vi "SCOPE_Measure.vi"(8 "error in (no error)":errorcluster, 9 "Data Cluster":T1 {"GUI Data Cluster"."SBR" format="%08b"}, 10 "Configuration Cluster":T3={"General"={"Config.ini"=path "", "Default Logging Path"=path ""}, "Hardware"={"Global T VAR"="", "Global B VAR"="", "VISAS"={"GEN COM"="", "SCOPE COM"="", "VNA COM"=""}, "Connected?"={"SCOPE"=FALSE, "GEN"=FALSE, "VNA"=FALSE}}, "Operation"={"Operation Mode"=enum."Idle-Off", "Status"="", "NewLog?"=FALSE, "OvenWarn"=FALSE, "Scope Settings"={"TimeBase"=0.0, "VerticalScale"=4.0, "Channel"=enum."Channel 2"}, "Gen Settings"={"Amplitude"=0.0, "Frequency"=0.0, "Offset"=0.0}}}) -> (0 "error out":errorcluster, 1 "Data Cluster out":T1 {"GUI Data Cluster"."SBR" format="%08b"}, 2 "Configuration Cluster Out":T3={"General"={"Config.ini"=path "", "Default Logging Path"=path ""}, "Hardware"={"Global T VAR"="", "Global B VAR"="", "VISAS"={"GEN COM"="", "SCOPE COM"="", "VNA COM"=""}, "Connected?"={"SCOPE"=FALSE, "GEN"=FALSE, "VNA"=FALSE}}, "Operation"={"Operation Mode"=enum."Idle-Off", "Status"="", "NewLog?"=FALSE, "OvenWarn"=FALSE, "Scope Settings"={"TimeBase"=0.0, "VerticalScale"=0.0, "Channel"=enum."Channel 2"}, "Gen Settings"={"Amplitude"=0.0, "Frequency"=0.0, "Offset"=0.0}}})   [LabVIEW 2021]
uses:
  Config_Cluster.ctl
  Mode_Enum.ctl
  Data_Cluster.ctl
  Measurement_Cluster.ctl
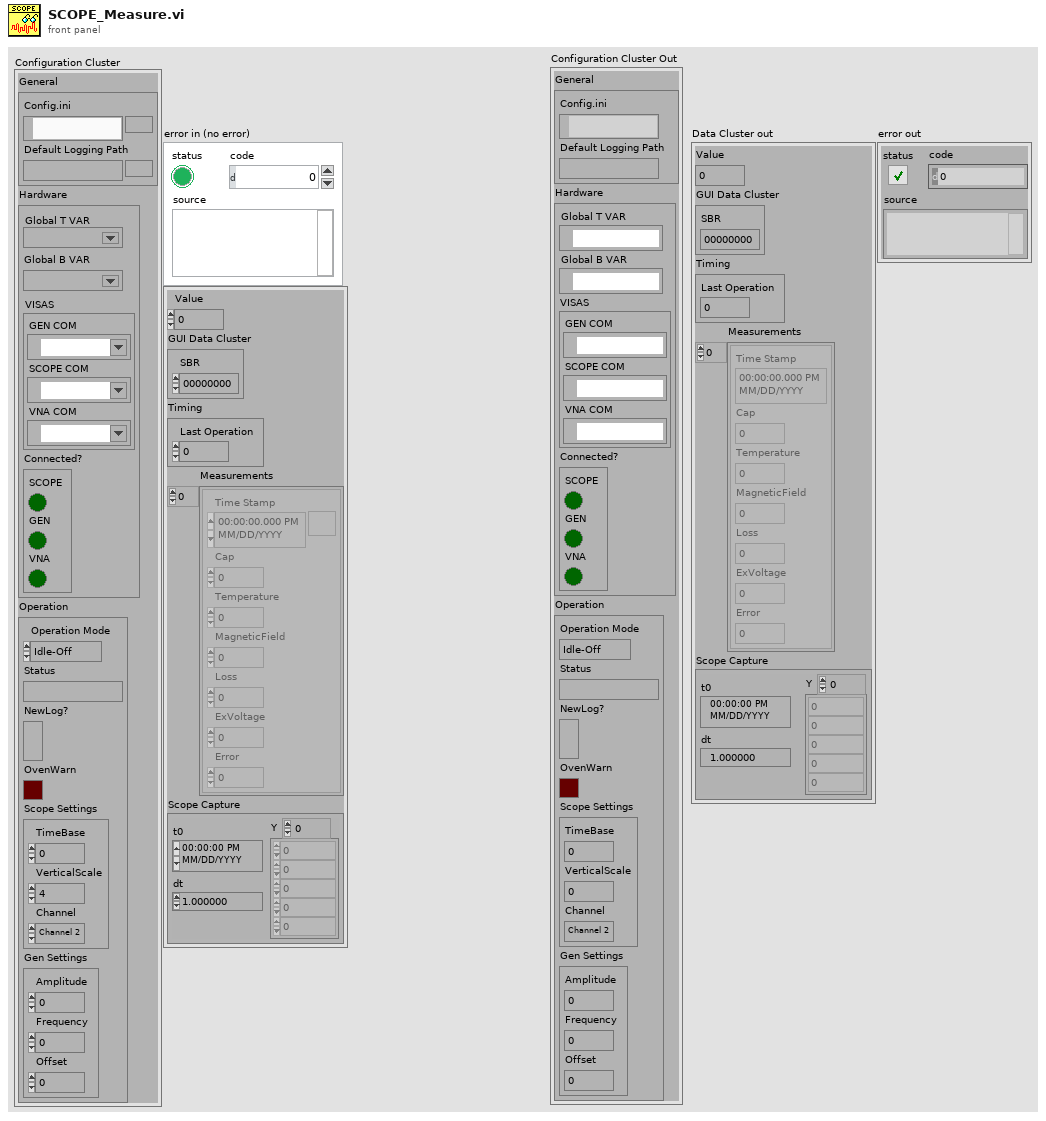
[diagram p1: front panel]
types:
  T1 = typedef "Data_Cluster.ctl" = cluster{"Value":dbl, "GUI Data Cluster":cluster{"SBR":u16}, "Timing":cluster{"Last Operation":dbl}, "Measurements":T2[], "Scope Capture":waveform(dbl)}
  T2 = typedef "Measurement_Cluster.ctl" = cluster{"Time Stamp":timestamp, "Cap":dbl, "Temperature":dbl, "MagneticField":dbl, "Loss":dbl, "ExVoltage":dbl, "Error":dbl}
  T3 = typedef "Config_Cluster.ctl" = cluster{"General":cluster{"Config.ini":path, "Default Logging Path":path}, "Hardware":cluster{"Global T VAR":refnum<k21>, "Global B VAR":refnum<k21>, "VISAS":cluster{"GEN COM":refnum<visa-resource-name>, "SCOPE COM":refnum<visa-resource-name>, "VNA COM":refnum<visa-resource-name>}, "Connected?":cluster{"SCOPE":bool, "GEN":bool, "VNA":bool}}, "Operation":cluster{"Operation Mode":T4, "Status":string, "NewLog?":bool, "OvenWarn":bool, "Scope Settings":cluster{"TimeBase":dbl, "VerticalScale":dbl, "Channel":enum16{"Channel 2", "Channel 1"}}, "Gen Settings":cluster{"Amplitude":dbl, "Frequency":dbl, "Offset":dbl}}}
  T4 = typedef "Mode_Enum.ctl" = enum16{"Logging", "Idle-Off", "Idle"}
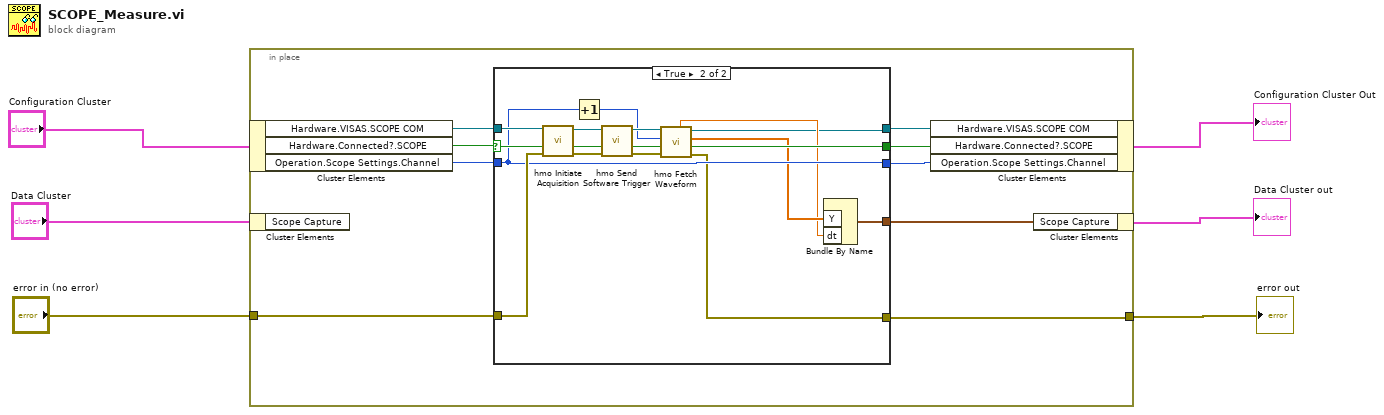
[diagram p0: block diagram]
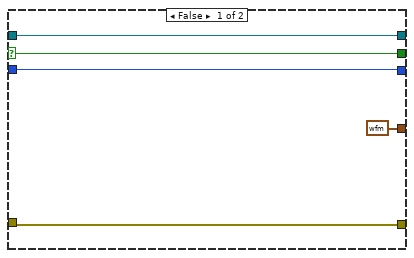
[diagram p2: hidden frame]
diagram:
  n1 = in-place {
    in-place-border: "error in (no error)" -> [w12]
    in-place-border: [w7] -> w1
    n2 = in-place-cluster #1("Configuration Cluster") -> ("Hardware.VISAS.SCOPE COM"=w13:refnum<visa-resource-name>, "Hardware.Connected?.SCOPE"=w15:bool, "Operation.Scope Settings.Channel"=w11:enum16{"Channel 2", "Channel 1"})
    n3 = in-place-cluster #2("Data Cluster") -> ()  [unwired: 1 out]
    n4 = case shown="True" w15 {
      selector: w15 -> [w20 w34]
      tunnel: [w20 w34] -> w14
      tunnel: w13 -> [w18 w33]
      tunnel: w12 -> [w16 w30]
      tunnel: w11 -> [w19 w26]
      tunnel: [w19 w26] -> w10
      tunnel: [w18 w22] -> w9
      tunnel: [waveform(dbl) {"t0"=timestamp(0 s since 1904-01-01), "dt"=1.0, "Y"=[]} w25] -> w8
      tunnel: [w16 w21] -> w7
      frame False {
      }
      frame True {
        n5 = call <instrlib>:"hmo Initiate Acquisition.vi"("error in (no error)"=w30, "VISA resource name"=w33) -> ("error out"=w31:errorcluster, "VISA resource name out"=w32:refnum<visa-resource-name>)  [unwired: 8 in]
        n6 = Increment(x=w26) -> (x+1=w27:enum16{"Channel 2", "Channel 1"})
        n7 = call <instrlib>:"hmo Send Software Trigger.vi"("error in (no error)"=w31, "VISA resource name"=w32) -> ("error out"=w28:errorcluster, "VISA resource name out"=w29:refnum<visa-resource-name>)  [unwired: 8 in]
        n8 = call <instrlib>:"hmo Fetch Waveform.vi"("error in (no error)"=w28, "Channel (1)"=w27, "VISA resource name"=w29) -> ("error out"=w21:errorcluster, "Waveform Array"=w24:dbl[], "VISA resource name out"=w22:refnum<visa-resource-name>, "X Increment"=w23:dbl)  [unwired: 3 in, 2 out]
        n9 = Bundle By Name("Y"=w24, "dt"=w23) -> (w25:waveform(dbl))  [unwired: 1 in]
      }
    }
    n10 = in-place-cluster #1("Hardware.VISAS.SCOPE COM"=w9, "Hardware.Connected?.SCOPE"=w14, "Operation.Scope Settings.Channel"=w10) -> (→"Configuration Cluster Out":T3)
    n11 = in-place-cluster #2("Scope Capture"=w8) -> (→"Data Cluster out":T1)
  }
  "error out" <- w1
